vi "resolve_VI_path_lua.vi"(5 "LuaVIEW reference":T1) -> (15 "error out":errorcluster)   [LabVIEW 2012]
doc: "Takes the name of a LuaVIEW-related VI and an optional toolkit subpath and resolves its location for the current runtime in a manner that works when built and when running in development mode. In development mode, the VI is assumed to be located in the directory of the toolkit/library/class extracted from the first part of the VI name, but converted to lower case. These are assumed to be subdirectories of the main LuaVIEW distribution directory. When built, the VI is assumed to be located in the application executable unless a minimal build is performed that leaves the LuaVIEW VIs outside the executable. In the latter case, the behaviour is the same as during development.\n\nMaking the toolkit/library/class part of the VI name is a convention followed by all LuaVIEW-related VIs. It mostly serves to avoid VI namespace collisions. As this function shows it can also be used to locate LuaVIEW-related VIs without needing to specify an absolute path.\nParameters:\nstr:VIname\n[str:subpath]\nResults:\nstr:path, path to VI"
uses:
  luaview/typedefs/t_LuaVIEW Reference.ctl
  luaview/subvis/private/LuaVIEW Pull (string).vi
  luaview/subvis/private/LuaVIEW Push (path).vi
  luaview/subvis/private/LuaVIEW Pull (path).vi
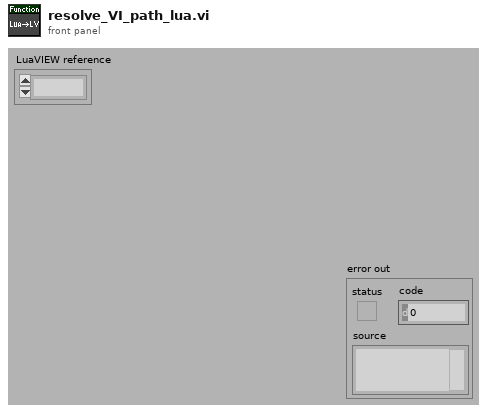
[diagram p1: front panel]
types:
  T1 = typedef "t_LuaVIEW Reference.ctl" = refnum<k1>
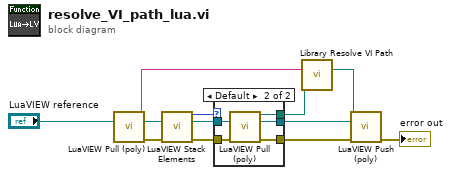
[diagram p0: block diagram]
diagram:
  n1 = call-poly "LuaVIEW Pull (poly).vi"("LuaVIEW reference in"="LuaVIEW reference") -> ("string"=w10:string, "LuaVIEW reference out"=w8:T1, "error out"=w9:errorcluster)  [unwired: 12 in]
  n2 = call "LuaVIEW Stack Elements.vi"("LuaVIEW reference in"=w8, "error in (no error)"=w9) -> ("elements"=w7:i32, "LuaVIEW reference out"=w5:T1, "error out"=w6:errorcluster)  [unwired: 11 in]
  n3 = case shown="Default" w7 {
    tunnel: w6 -> [w13 w18]
    tunnel: w5 -> [w14 w19]
    tunnel: [w14 w16] -> w4
    tunnel: [w13 w17] -> w3
    tunnel: [_ w15] -> w2
    frame 0 {
    }
    frame Default {
      n4 = call-poly "LuaVIEW Pull (poly).vi"("LuaVIEW reference in"=w19, "error in (no error)"=w18) -> ("path"=w15:path, "LuaVIEW reference out"=w16:T1, "error out"=w17:errorcluster)  [unwired: 11 in]
    }
  }
  n5 = call "Library Resolve VI Path.vi"("VI name"=w10, "sub path of toolkit (none)"=w2) -> ("VI path"=w1:path)  [unwired: 13 in]
  n6 = call-poly "LuaVIEW Push (poly).vi"("path"=w1, "LuaVIEW reference in"=w4, "error in (no error)"=w3) -> ("error out"=→"error out":errorcluster)  [unwired: 11 in, 1 out]
